vi "niDTS WLAN Dut Tx Post Initiate.vi"(0 "Dut Handle in":T1, 11 "error in (no error)":errorcluster) -> (4 "Dut Handle out":T1, 15 "error out":errorcluster)   [LabVIEW 2015, in "niDTS WLAN.lvlib"]
uses:
  niDTS WLAN.lvlib
  Framework/Dut/Includes/niDTS Dut INC Handle.ctl
  Framework/Dut/Objects/BASE_class/niDTS Dut.lvclass
  Includes/niDTS WLAN Dut INC Handle.ctl
  Objects/BASE_class/niDTS WLAN Dut.lvclass
  Framework/niDTS Framework.lvlib
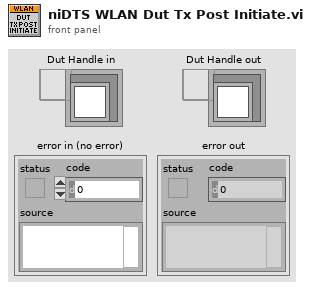
[diagram p1: front panel]
types:
  T1 = typedef "niDTS Framework.lvlib/niDTS Dut INC Handle.ctl" = refnum<data-value>
  T2 = typedef "niDTS WLAN.lvlib/niDTS WLAN Dut INC Handle.ctl" = refnum<data-value>
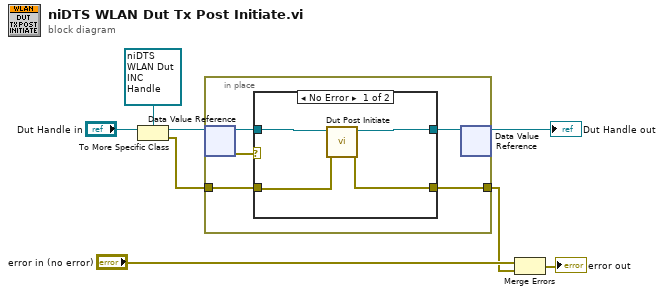
[diagram p0: block diagram]
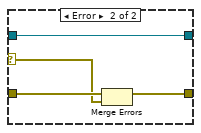
[diagram p2: hidden frame]
diagram:
  n1 = To More Specific Class(target class=T2 refnum ("WLAN Dut Handle"), reference="Dut Handle in") -> (specific class reference=w5:T2, error out=w4:errorcluster)  [unwired: 1 in]
  n2 = in-place {
    in-place-border: w4 -> [w10]
    in-place-border: [w9] -> w2
    n3 = in-place-dvr #1(w5) -> (w12:refnum<class "niDTS WLAN Dut.lvclass">, w13:errorcluster)
    n4 = case shown="No Error" w13 {
      selector: w13 -> [_ w19]
      tunnel: w12 -> [w17 w21]
      tunnel: [w16 w21] -> w11
      tunnel: w10 -> [w14 w20]
      tunnel: [w15 w18] -> w9
      frame No Error {
        n5 = call-dynamic "Dut Post Initiate.vi"("error in (no error)"=w14, "niDTS Dut in"=w17) -> ("error out"=w15:errorcluster, "niDTS Dut out"=w16:refnum<class "niDTS WLAN Dut.lvclass">)  [unwired: 8 in]
      }
      frame Error {
        n6 = Merge Errors(w20, w19) -> (w18:errorcluster)
      }
    }
    n7 = in-place-dvr #1(w11) -> (→"Dut Handle out":T2)  [unwired: 1 out]
  }
  n8 = Merge Errors("error in (no error)", w2) -> (→"error out":errorcluster)
